vi "SVT Frequency Response (Mag-Phase).vi"   [LabVIEW 2017]
doc: "Computes the frequency response and coherence based on <B>stimulus signal X [EUx]</B> and <B>response signal Y [EUy]</B>. Results are returned as <B>magnitude [dB EUy/EUx]</B>, <B>phase [degrees]</B>, and <B>coherence</B>."
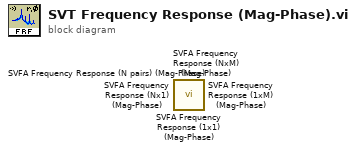
[diagram p0: block diagram]
diagram:
  n1 = call <vilib>:"SVFA Frequency Response (1x1) (Mag-Phase).vi"() -> ()  [unwired: 11 in, 9 out]
  n2 = call <vilib>:"SVFA Frequency Response (NxM) (Mag-Phase).vi"() -> ()  [unwired: 11 in, 9 out]
  n3 = call <vilib>:"SVFA Frequency Response (Nx1) (Mag-Phase).vi"() -> ()  [unwired: 11 in, 9 out]
  n4 = call <vilib>:"SVFA Frequency Response (1xM) (Mag-Phase).vi"() -> ()  [unwired: 11 in, 9 out]
  n5 = call <vilib>:"SVFA Frequency Response (N pairs) (Mag-Phase).vi"() -> ()  [unwired: 11 in, 9 out]
